vi "Create.vi"() -> (8 "FM Sweep":refnum<class "FM Sweep.lvclass">)   [LabVIEW 2020, in "FM Sweep.lvclass"]
uses:
  FM Sweep.lvclass
  FM Sweep.lvclass/FM Sweep.ctl
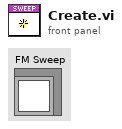
[diagram p1: front panel]
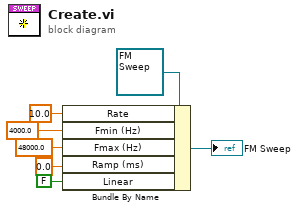
[diagram p0: block diagram]
diagram:
  n1 = Bundle By Name(cluster=refnum<class "FM Sweep.lvclass"> refnum ("FM Sweep"), "Rate"=10.0 ("Serialized.Rate"), "Fmin (Hz)"=4000.0 ("Serialized.Fmin (Hz)"), "Fmax (Hz)"=48000.0 ("Serialized.Fmax (Hz)"), "Ramp (ms)"=0.0 ("Serialized.Ramp (ms)"), "Linear"=FALSE ("Serialized.Linear")) -> (→"FM Sweep":refnum<class "FM Sweep.lvclass">)
